vi "Autonics_Hall_GMR_Vector.vi"() -> ()   [LabVIEW 2018]
uses:
  <vilib>/Platform/NI_3dgraph.lvlib
  <vilib>/Utility/file.llb/Write To Spreadsheet File (DBL).vi
  <vilib>/DAQmx/create/channels.llb/DAQmx Create Channel (DO-Digital Output).vi
  <vilib>/DAQmx/write.llb/DAQmx Write (Digital 1D Bool 1Chan 1Samp).vi
  <vilib>/DAQmx/read.llb/DAQmx Read (Analog 2D DBL NChan NSamp).vi
  <vilib>/DAQmx/configure/timing.llb/DAQmx Timing (Sample Clock).vi
  <vilib>/DAQmx/create/channels.llb/DAQmx Create Channel (AI-Voltage-Basic).vi
  <resource>/objmgr/daqmx.rc
  <vilib>/Math Plots/3D Math Plots/3D Quiver/3D Quiver Datatype/3D Quiver Datatype.lvclass
  <vilib>/Math Plots/3D Math Plots/3D Quiver/3D Quiver Datatype/Public/Plot Helper (Vector).vi
  <vilib>/Analysis/Matrix/NI_Matrix.lvlib
  <vilib>/Utility/file.llb/Read From Spreadsheet File (DBL).vi
  <vilib>/Analysis/Matrix/Numeric/Multiply/Multiply - R,RM.vi
  <vilib>/Analysis/Matrix/Numeric/Multiply/Multiply - RM,R.vi
  <vilib>/Math Plots/2D Math Plots/2D Feather/2D Feather Datatype/2D Feather Datatype.lvclass
  <vilib>/Math Plots/2D Math Plots/2D Feather/2D Feather Datatype/Public/Plot Helper (Vector).vi
  <vilib>/Instr/_visa.llb/VISA Configure Serial Port (Instr).vi
  <vilib>/Math Plots/3D Math Plots/3D Quiver/3D Quiver XCtrl/3D Quiver.xctl
  <vilib>/Math Plots/2D Math Plots/2D Feather/2D Feather XCtrl/2D Feather.xctl
panel:
  out "2D Feather":refnum<class "2D Plot Datatype.lvclass">[](xcontrol)
  in  "GMR":refnum<k7>(container)
  in  "Z Length":dbl=2.0
  out "X Length":dbl=50.0
  out "X_Z_Scale":sgl=111.11112
  in  "Invert ?":bool
  out "Time Step":u32
  in  "Open":bool
  out "3D Vector":refnum<class "3D Plot Datatype.lvclass">[](xcontrol)
  in  "Scan Distance":dbl=50.0
  in  "Multiplier":dbl=10.0
  in  "Save Button":bool
  in  "No Save":bool
  in  "Save/Open Link":path
  in  "ViewMode":i32(ring) items=["cwViewXYPlane", "cwViewXZPlane", "cwViewYZPlane", "cwViewUserDefined"]
  in  "Back data":bool
  in  "Data Type":u16(ring) items=["Normal", "dX", "dY"]
  in  "Scan Channel":fxp<+,8,8>
  in  "Scan Channel Control":tag="Dev3/port0/line0:7"
  in  "Sampling Rate(Hz)":dbl=15000.0
  in  "Samples per Channels":i32=1000
  in  "Min Volts":dbl=-10.0 format="%0.2f"
  in  "Max Volts":dbl=10.0 format="%0.2f"
  in  "Channels":tag="Dev3/ai0:63"
  in  "Scan Step (mm)":dbl=1.0
  in  "Scan":bool
  in  "Plot style":i32(ring)=5 items=["cwLine"=1, "cwPoint"=2, "cwLinePoint"=3, "cwHiddenLine"=4, "cwSurface"=5, "cwSurfaceLine"=6, "cwSurfaceNormal"=7, "cwContourLine"=8, "cwSurfaceContour"=9]
  in  "Hall":refnum<k7>(container)
  in  "Flow control":u16(ring) items=["None", "XON/XOFF", "RTS/CTS", "XON/XOFF & RTS/CTS", "DTR/DSR", "XON/XOFF & DTR/DSR"]
  in  "Stop bits":u16(ring)=10 items=["1.0"=10, "1.5"=15, "2.0"=20]
  in  "Parity":dbl
  in  "Data bits":u16=8 min=5 max=8 step=1
  in  "Baud Rate":u32=57600
  in  "COM Port":refnum<visa-resource-name>="COM3"
  in  "Travel per Pulse (mm)":dbl=0.002
  in  "Speed (mm/s)":dbl=5.0
  out "Current  Position (mm)":dbl format="%#_4g"
  in  "Move Distance (mm)":dbl=1.0
  in  "Stop Scan":bool
  in  "Stop":bool
  in  "Home":bool
  in  "Right":bool
  in  "Left":bool
  # "SCANER CONTROL"
  # "CRACKS INSPECTION"
  # "COM Setting"
  # "CHANNELS"
  # "TIMING"
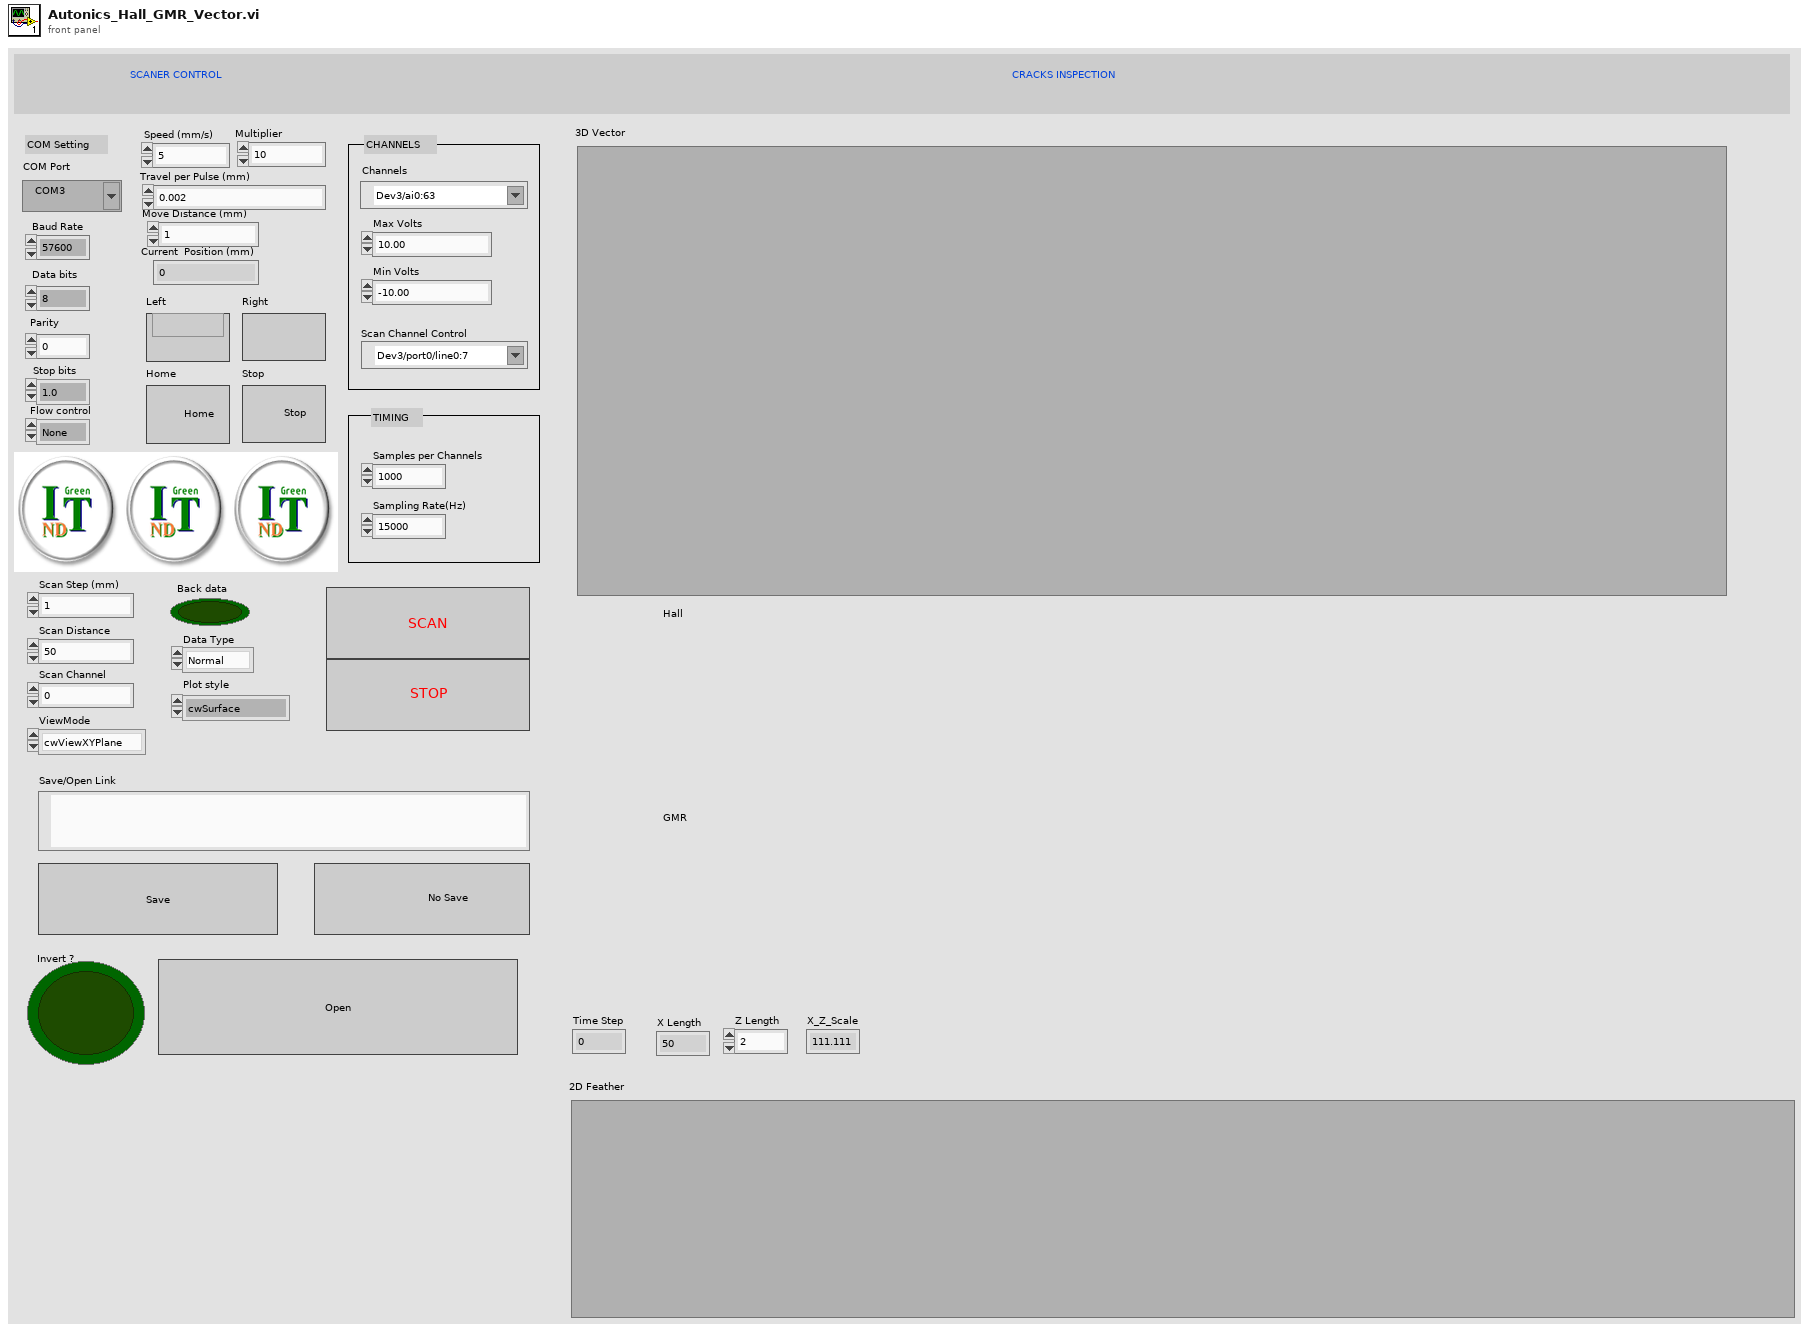
[diagram p1: front panel]
types:
  T1 = typedef "NI_Matrix.lvlib/RealMatrix.ctl" = dbl[][]
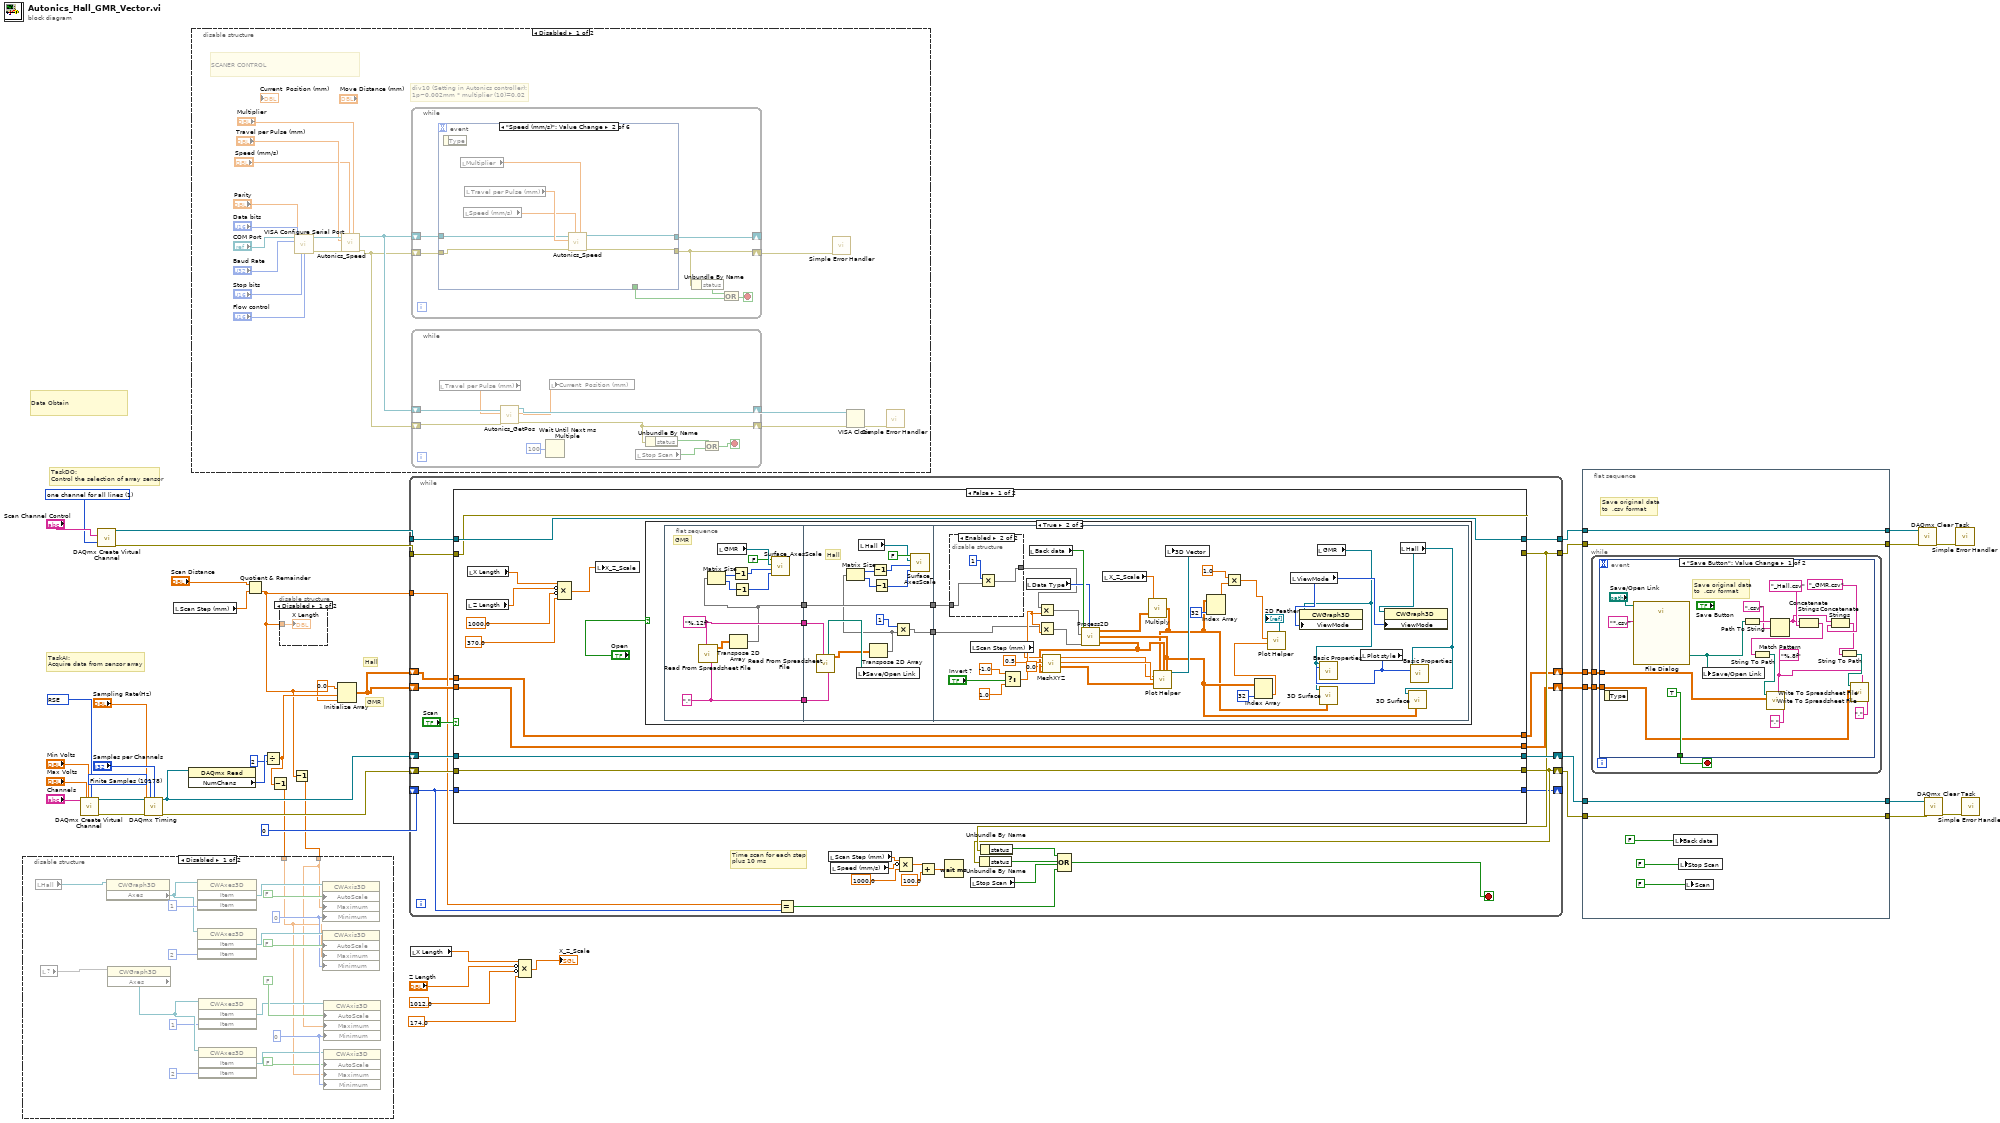
[diagram p0: block diagram]
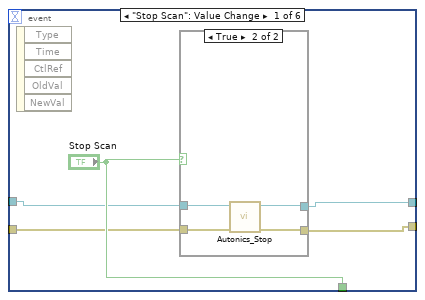
[diagram p4: hidden frame]
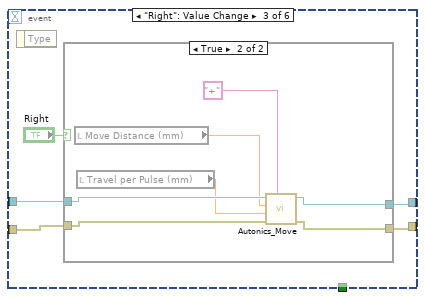
[diagram p6: hidden frame]
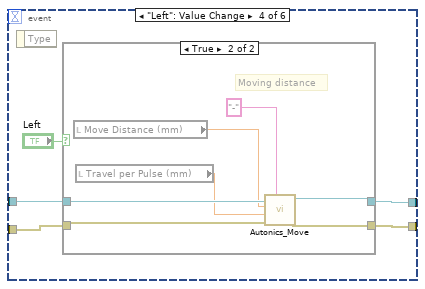
[diagram p8: hidden frame]
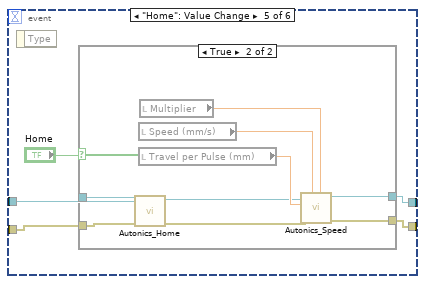
[diagram p10: hidden frame]
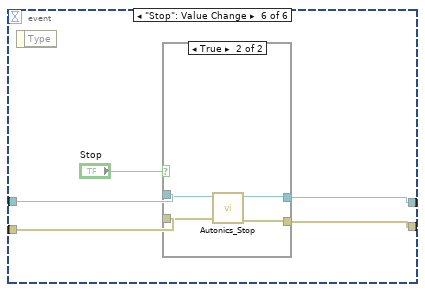
[diagram p12: hidden frame]
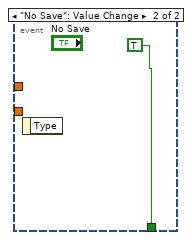
[diagram p15: hidden frame]
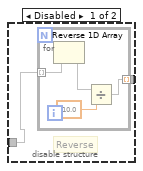
[diagram p17: hidden frame]
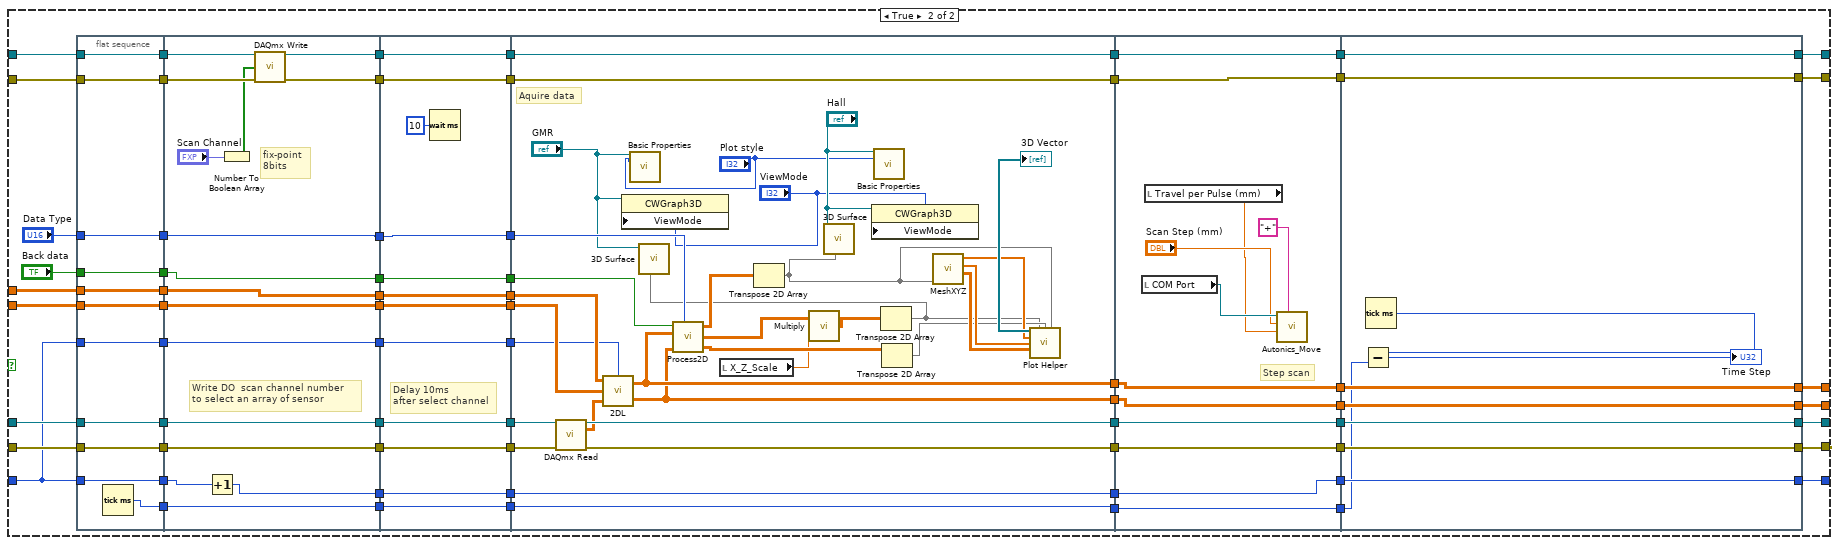
[diagram p18: hidden frame]
diagram:
  w20 = 10083 items=["default"=-1, "RSE"=10083, "NRSE"=10078, "Differential"=10106, "Pseudodifferential"=12529] ("input terminal configuration")
  w28 = 1 items=["one channel for each line", "one channel for all lines"] ("line grouping")
  w34 = 10178 items=["Finite Samples"=10178, "Continuous Samples"=10123, "Hardware Timed Single Point"=12522] ("sample mode")
  # "GMR"
  # "Hall"
  # "TaskAI:\nAcquire data from sensor array"
  # "TaskDO: \nControl the selection of array sensor"
  # "Data Obtain"
  n1 = call-poly <vilib>:"DAQmx Create Virtual Channel.vi"("maximum value"="Max Volts", "minimum value"="Min Volts", "input terminal configuration"=w20, "physical channels"="Channels") -> ("task out"=w43:refnum<k21>, "error out"=w42:errorcluster)  [unwired: 10 in]
  n2 = call-poly <vilib>:"DAQmx Create Virtual Channel.vi"("lines"="Scan Channel Control", "line grouping"=w28) -> ("task out"=w27:refnum<k21>, "error out"=w26:errorcluster)  [unwired: 12 in]
  n3 = call-poly <vilib>:"DAQmx Timing.vi"("task/channels in"=w43, "sample mode"=w34, "samples per channel"="Samples per Channels", "rate"="Sampling Rate(Hz)", "error in"=w42) -> ("task out"=w18:refnum<k21>, "error out"=w36:errorcluster)  [unwired: 9 in]
  n4 = local read "Scan Step (mm)"() -> (w17:dbl)
  n5 = property class="DAQmx Read"(reference=w18) -> ("NumChans"=w13:u32)  [unwired: 1 in, 2 out]
  n6 = disable-structure shown="Disabled" {
    frame Disabled {
      # "div10 (Setting in Autonics controller):\n1p~0.002mm * multiplier (10)=0.02"
      # "SCANER CONTROL"
      n7 = call-poly "VISA Configure Serial Port"("VISA resource name"="COM Port", "baud rate (9600)"="Baud Rate", "data bits (8)"="Data bits", "parity (0:none)"="Parity", "stop bits (10: 1 bit)"="Stop bits", "flow control (0:none)"="Flow control") -> ("VISA resource name out"=w48:refnum<visa-resource-name>, "error out"=w47:errorcluster)  [unwired: 8 in]
      n8 = call "Autonics_Speed.vi"("Multiplier"="Multiplier", "Speed (mm/s)"="Speed (mm/s)", "error in (no error)"=w47, "Travel per  Pulse"="Travel per Pulse (mm)", "VISA resource name"=w48) -> ("error out"=w49:errorcluster, "VISA resource name out"=w50:refnum<visa-resource-name>)  [unwired: 5 in]
      n9 = while {
        shift-right: [w77] -> _
        shift-left: w50 -> [w76]
        shift-right: [w73] -> w53
        shift-left: w49 -> [w75]
        stop <- w72 stop-if-true
        n10 = event shown="[1] \"Speed (mm/s)\": Value Change" {
          selector: _ -> [_ _ _ _ _ _]
          dyn-events: _ -> [_ _ _ _ _ _]
          timeout: _ -> [_ _ _ _ _ _]
          tunnel: w76 -> [w81 w94 w98 w112 w128 w142]
          tunnel: w75 -> [w80 w93 w97 w111 w127 w141]
          tunnel: [w79 w92 w100 w114 w125 w144] -> w77
          tunnel: [w78 w91 w99 w113 w124 w143] -> w73
          tunnel: ["Stop Scan" _ _ _ _ _] -> w71
          event "Stop Scan": Value Change {
            n11 = event-data() -> ()  [unwired: 1 in, 5 out]
            n12 = case shown="True" "Stop Scan" {
              tunnel: [w84 w87] -> w79
              tunnel: [w83 w88] -> w78
              tunnel: w81 -> [w84 w86]
              tunnel: w80 -> [w83 w85]
              frame False {
              }
              frame True {
                n13 = call "Autonics_Stop.vi"("error in (no error)"=w85, "VISA resource name"=w86) -> ("error out"=w88:errorcluster, "VISA resource name out"=w87:refnum<visa-resource-name>)  [unwired: 8 in]
              }
            }
          }
          event "Speed (mm/s)": Value Change {
            n14 = event-data() -> ()  [unwired: 1 in, 1 out]
            n15 = local read "Multiplier"() -> (w89:dbl)
            n16 = local read "Speed (mm/s)"() -> (w90:dbl)
            n17 = local read "Travel per Pulse (mm)"() -> (w95:dbl)
            n18 = call "Autonics_Speed.vi"("Multiplier"=w89, "Speed (mm/s)"=w90, "error in (no error)"=w93, "Travel per  Pulse"=w95, "VISA resource name"=w94) -> ("error out"=w91:errorcluster, "VISA resource name out"=w92:refnum<visa-resource-name>)  [unwired: 5 in]
          }
          event "Right": Value Change {
            n19 = event-data() -> ()  [unwired: 1 in, 1 out]
            n20 = case shown="True" "Right" {
              tunnel: [w101 w107] -> w100
              tunnel: [w102 w106] -> w99
              tunnel: w98 -> [w101 w109]
              tunnel: w97 -> [w102 w108]
              frame False {
              }
              frame True {
                n21 = local read "Move Distance (mm)"() -> (w105:dbl)
                n22 = local read "Travel per Pulse (mm)"() -> (w104:dbl)
                n23 = call "Autonics_Move.vi"("Direction (+)"="+", "error in (no error)"=w108, "Travel per Pulse (mm)"=w104, "Move Distance (mm)"=w105, "VISA resource name"=w109) -> ("error out"=w106:errorcluster, "VISA resource name out"=w107:refnum<visa-resource-name>)  [unwired: 5 in]
              }
            }
          }
          event "Left": Value Change {
            n24 = event-data() -> ()  [unwired: 1 in, 1 out]
            n25 = case shown="True" "Left" {
              tunnel: [w116 w121] -> w114
              tunnel: [w115 w120] -> w113
              tunnel: w112 -> [w116 w123]
              tunnel: w111 -> [w115 w122]
              frame False {
              }
              frame True {
                # "Moving distance"
                n26 = local read "Move Distance (mm)"() -> (w118:dbl)
                n27 = local read "Travel per Pulse (mm)"() -> (w117:dbl)
                n28 = call "Autonics_Move.vi"("Direction (+)"="-", "error in (no error)"=w122, "Travel per Pulse (mm)"=w117, "Move Distance (mm)"=w118, "VISA resource name"=w123) -> ("error out"=w120:errorcluster, "VISA resource name out"=w121:refnum<visa-resource-name>)  [unwired: 5 in]
              }
            }
          }
          event "Home": Value Change {
            n29 = event-data() -> ()  [unwired: 1 in, 1 out]
            n30 = case shown="True" "Home" {
              tunnel: [w130 w132] -> w125
              tunnel: [w129 w131] -> w124
              tunnel: w128 -> [w130 w139]
              tunnel: w127 -> [w129 w138]
              frame False {
              }
              frame True {
                n31 = call "Autonics_Home.vi"("error in (no error)"=w138, "VISA resource name"=w139) -> ("error out"=w133:errorcluster, "VISA resource name out"=w134:refnum<visa-resource-name>)  [unwired: 8 in]
                n32 = local read "Speed (mm/s)"() -> (w136:dbl)
                n33 = local read "Travel per Pulse (mm)"() -> (w137:dbl)
                n34 = local read "Multiplier"() -> (w135:dbl)
                n35 = call "Autonics_Speed.vi"("Multiplier"=w135, "Speed (mm/s)"=w136, "error in (no error)"=w133, "Travel per  Pulse"=w137, "VISA resource name"=w134) -> ("error out"=w131:errorcluster, "VISA resource name out"=w132:refnum<visa-resource-name>)  [unwired: 5 in]
              }
            }
          }
          event "Stop": Value Change {
            n36 = event-data() -> ()  [unwired: 1 in, 1 out]
            n37 = case shown="True" "Stop" {
              tunnel: [w146 w147] -> w144
              tunnel: [w145 w150] -> w143
              tunnel: w142 -> [w146 w149]
              tunnel: w141 -> [w145 w148]
              frame False {
              }
              frame True {
                n38 = call "Autonics_Stop.vi"("error in (no error)"=w148, "VISA resource name"=w149) -> ("error out"=w150:errorcluster, "VISA resource name out"=w147:refnum<visa-resource-name>)  [unwired: 8 in]
              }
            }
          }
        }
        n39 = Unbundle By Name(w73) -> ("status"=w74:bool)
        n40 = Compound Arithmetic op=OR(w74, w71) -> (w72:bool)
      }
      n41 = while {
        shift-right: [w64] -> w52
        shift-left: w50 -> [w66]
        shift-right: [w63] -> w51
        shift-left: w49 -> [w65]
        stop <- w67 stop-if-true
        n42 = local read "Travel per Pulse (mm)"() -> (w62:dbl)
        n43 = call "Autonics_GetPos.vi"("error in (no error)"=w65, "Travel per Pulse (mm)"=w62, "VISA resource name"=w66) -> ("error out"=w63:errorcluster, "Current  Position (mm)"=w61:dbl, "VISA resource name out"=w64:refnum<visa-resource-name>)  [unwired: 6 in]
        n44 = Wait Until Next ms Multiple(millisecond multiple=u32 100) -> ()  [unwired: 1 out]
        n45 = local write "Current  Position (mm)"(w61) -> ()
        n46 = local read "Stop Scan"() -> (w68:bool)
        n47 = Unbundle By Name(w63) -> ("status"=w69:bool)
        n48 = Compound Arithmetic op=OR(w69, w68) -> (w67:bool)
      }
      n49 = call <vilib>:"Simple Error Handler.vi"("error in (no error)"=w53) -> ()  [unwired: 4 in, 5 out]
      n50 = VISA Close(VISA resource name=w52, error in (no error)=w51) -> (error out=w56:errorcluster)
      n51 = call <vilib>:"Simple Error Handler.vi"("error in (no error)"=w56) -> ()  [unwired: 4 in, 5 out]
    }
    frame Enabled {
    }
  }
  n52 = Quotient & Remainder(x="Scan Distance", y=w17) -> (floor(x/y)=w7:dbl)  [unwired: 1 out]
  n53 = Divide(x=w13, y=u32 2) -> (x/y=w9:dbl)
  n54 = Decrement(x=w9) -> (x-1=w10:dbl)
  n55 = disable-structure shown="Disabled" {
    disable-tunnel: w7 -> [w151 _]
    frame Disabled {
      "X Length" <- w151
    }
    frame Enabled {
    }
  }
  n56 = Decrement(x=w7) -> (x-1=w8:dbl)
  n57 = disable-structure shown="Disabled" {
    disable-tunnel: w10 -> [w153 _]
    disable-tunnel: w8 -> [w152 _]
    frame Disabled {
      w162 = 0
      w163 = 0
      n58 = local read "Hall"() -> (w171:refnum<k7>)
      n59 = local read item#-1() -> (w154)
      n60 = property class="CWGraph3D"(reference=w171) -> ("Axes"=w164:refnum<k7>)  [unwired: 1 in, 2 out]
      n61 = property class="CWGraph3D"(reference=w154) -> ("Axes"=w161:refnum<k7>)  [unwired: 1 in, 2 out]
      n62 = invoke class="CWAxes3D" method="Item"(reference=w164, "Item"=1) -> ("Item"=w170:refnum<k7>)  [unwired: 2 in, 3 out]
      n63 = invoke class="CWAxes3D" method="Item"(reference=w164, "Item"=2) -> ("Item"=w165:refnum<k7>)  [unwired: 2 in, 3 out]
      n64 = invoke class="CWAxes3D" method="Item"(reference=w161, "Item"=1) -> ("Item"=w155:refnum<k7>)  [unwired: 2 in, 3 out]
      n65 = invoke class="CWAxes3D" method="Item"(reference=w161, "Item"=2) -> ("Item"=w160:refnum<k7>)  [unwired: 2 in, 3 out]
      n66 = property class="CWAxis3D"(reference=w170, "AutoScale"=FALSE, "Maximum"=w152, "Minimum"=w163) -> ()  [unwired: 1 in, 2 out]
      n67 = property class="CWAxis3D"(reference=w165, "AutoScale"=FALSE, "Maximum"=w153, "Minimum"=w163) -> ()  [unwired: 1 in, 2 out]
      n68 = property class="CWAxis3D"(reference=w155, "AutoScale"=FALSE, "Maximum"=w152, "Minimum"=w162) -> ()  [unwired: 1 in, 2 out]
      n69 = property class="CWAxis3D"(reference=w160, "AutoScale"=FALSE, "Maximum"=w153, "Minimum"=w162) -> ()  [unwired: 1 in, 2 out]
    }
    frame Enabled {
    }
  }
  n70 = Initialize Array(0.0 ("element"), w9, w7) -> (w14:dbl[][])
  n71 = while {
    shift-right: [w172] -> w1
    shift-left: w14 -> [w197]
    shift-right: [w195] -> w33
    shift-left: w18 -> [w196]
    shift-right: [w187] -> w31
    shift-left: w36 -> [w198]
    tunnel: w27 -> [w191]
    tunnel: w26 -> [w190]
    tunnel: [w189] -> w24
    tunnel: [w188] -> w23
    shift-right: [w178] -> _
    shift-left: 0 -> [w176]
    tunnel: w7 -> [w177]
    shift-right: [w173] -> w11
    shift-left: w14 -> [w174]
    stop <- w194 stop-if-true
    # "Time scan for each step\nplus 10 ms"
    n72 = case shown="False" "Scan" {
      tunnel: w196 -> [w211 w348]
      tunnel: w198 -> [w210 w347]
      tunnel: w197 -> [w206 w346]
      tunnel: [w211 w343] -> w195
      tunnel: [w210 w342] -> w187
      tunnel: [w205 w309] -> w173
      tunnel: w191 -> [w209 w341]
      tunnel: w190 -> [w208 w340]
      tunnel: [w209 w337] -> w189
      tunnel: [w208 w336] -> w188
      tunnel: [w207 w319] -> w178
      tunnel: w176 -> [w207 w312]
      tunnel: w174 -> [w205 w313]
      tunnel: [w206 w307] -> w172
      frame False {
        n73 = local read "Z Length"() -> (w203:dbl)
        n74 = local read "X Length"() -> (w202:dbl)
        n75 = Compound Arithmetic op=MULTIPLY(w202, invert w203, invert 1000.0 ("value"), 370.0 ("value")) -> (w199:dbl)
        n76 = local write "X_Z_Scale"(w199) -> ()
        n77 = case shown="True" "Open" {
          frame False {
          }
          frame True {
            n78 = flat-sequence {
              tunnel: [w218] -> w215
              tunnel: [w226] -> w213
              tunnel: [w225] -> w212
              tunnel: [w240] -> w216
              tunnel: w215 -> [w240]
              tunnel: [w230] -> w214
              tunnel: w213 -> [w239]
              tunnel: w212 -> [w238]
              tunnel: w216 -> [w257]
              tunnel: w214 -> [w246]
              frame #0 {
                w226 = "," ("delimiter (\\t)")
                w225 = "%.12f" ("format (%.3f)")
                # "GMR"
                n79 = call-poly <vilib>:"Read From Spreadsheet File.vi"("delimiter (\\t)"=w226, "format (%.3f)"=w225) -> ("all rows"=w217:dbl[][])  [unwired: 5 in, 4 out]
                n80 = local read "GMR"() -> (w221:refnum<k7>)
                n81 = Transpose 2D Array(2D array=w217) -> (transposed array=w218:dbl[][])
                n82 = Matrix Size(0:w218) -> (1:w219:i32, 2:w223:i32)
                n83 = Decrement(x=w219) -> (x-1=w222:i32)
                n84 = Decrement(x=w223) -> (x-1=w224:i32)
                n85 = call "Surface_AxesScale.vi"("Y-axis Max"=w224, "X-axis max"=w222, "3D Surface"=w221, "Auto Scale"=FALSE) -> ()  [unwired: 8 in]
              }
              frame #1 {
                # "Hall"
                n86 = call-poly <vilib>:"Read From Spreadsheet File.vi"("delimiter (\\t)"=w239, "format (%.3f)"=w238) -> ("all rows"=w228:dbl[][], "new file path (Not A Path if cancelled)"=w237:path)  [unwired: 5 in, 3 out]
                n87 = local write "Save/Open Link"(w237) -> ()
                n88 = local read "Hall"() -> (w234:refnum<k7>)
                n89 = Transpose 2D Array(2D array=w228) -> (transposed array=w227:dbl[][])
                n90 = Matrix Size(0:w227) -> (1:w236:i32, 2:w232:i32)
                n91 = Decrement(x=w236) -> (x-1=w233:i32)
                n92 = Decrement(x=w232) -> (x-1=w231:i32)
                n93 = Multiply(x=1, y=w227) -> (x*y=w230:dbl[][])
                n94 = call "Surface_AxesScale.vi"("Y-axis Max"=w231, "X-axis max"=w233, "3D Surface"=w234, "Auto Scale"=FALSE) -> ()  [unwired: 8 in]
              }
              frame #2 {
                n95 = disable-structure shown="Enabled" {
                  disable-tunnel: w257 -> [w276 w283]
                  disable-tunnel: [w275 w282] -> w247
                  frame Disabled {
                    # "Reverse"
                    n96 = for {
                      tunnel: w276 -> [w280] mode=indexing
                      tunnel: [w277] -> w275 mode=indexing
                      n97 = Reverse 1D Array(array=w280) -> (reversed array=w278:dbl[])
                      n98 = Divide(x=w278, y=-10.0 ("t")) -> (x/y=w277:dbl[])
                    }
                  }
                  frame Enabled {
                    n99 = Multiply(x=1, y=w283) -> (x*y=w282:dbl[][])
                  }
                }
                n100 = local read "Scan Step (mm)"() -> (w260:dbl)
                n101 = Select(t=-1.0, s="Invert ?", f=1.0) -> (s? t:f=w268:dbl)
                n102 = local read "Data Type"() -> (w261:u16)
                n103 = local read "Back data"() -> (w262:bool)
                n104 = Multiply(x=w247, y=w268) -> (x*y=w255:dbl[][])
                n105 = Multiply(x=w246, y=w268) -> (x*y=w267:dbl[][])
                n106 = call "Process2D.vi"("Back Data"=w262, "Matrix X"=w255, "Matrix Y"=w267, "Data Type"=w261) -> ("Out Matrix X"=w244:T1, "Out Matrix Y"=w245:T1, "Out Matrix Z (zeros)"=w256:T1)  [unwired: 1 in]
                n107 = call "MeshXYZ.vi"("Input Matrix)"=w256, "Z- Lift-off"=0.0, "del Y"=0.5, "del X"=w260) -> ("Mesh Z (Matrix)"=w243:dbl[][], "Mesh Y (Array)"=w274:dbl[], "Mesh X (Array)"=w273:dbl[])  [unwired: 5 in]
                n108 = local read "X_Z_Scale"() -> (w258:sgl)
                n109 = call-poly <vilib>:"Multiply.vi"("Real Matrix A"=w244, "Real Scalar c"=w258) -> ("c * A"=w242:T1)
                n110 = call-poly <vilib>:"Plot Helper.vi"("Nx matrix"=w242, "Ny matrix"=w256, "Nz matrix"=w245, "x vector"=w273, "y vector"=w274, "z matrix"=w243) -> ("3D Plot lvclass Array out"=w272:refnum<class "3D Plot Datatype.lvclass">[])  [unwired: 3 in, 6 out]
                n111 = local write "3D Vector"(w272) -> ()
                n112 = Index Array(array=w242, index (col)=32 ("disabled index (col)")) -> (element=w249:dbl[])  [unwired: 1 in]
                n113 = Multiply(x=1.0, y=w249) -> (x*y=w248:dbl[])
                n114 = Index Array(array=w245, index (col)=32 ("disabled index (col)")) -> (element=w251:dbl[])  [unwired: 1 in]
                n115 = call-poly <vilib>:"Plot Helper.vi"("y vector"=w251, "x vector"=w248) -> ("2D Plot Class Obj Array out"=→"2D Feather":refnum<class "2D Plot Datatype.lvclass">[])  [unwired: 2 in, 7 out]
                n116 = local read "ViewMode"() -> (w265:i32)
                n117 = local read "GMR"() -> (w263:refnum<k7>)
                n118 = property class="CWGraph3D"(reference=w263, "ViewMode"=w265) -> ()  [unwired: 1 in, 2 out]
                n119 = call <vilib>:"3D Surface.vi"("z matrix"=w242, "3D graph"=w263) -> ()  [unwired: 8 in, 2 out]
                n120 = local read "Plot style"() -> (w266:i32)
                n121 = call <vilib>:"Basic Properties.vi"("3D graph"=w263, "plot style"=w266) -> ()  [unwired: 12 in, 2 out]
                n122 = local read "Hall"() -> (w264:refnum<k7>)
                n123 = property class="CWGraph3D"(reference=w264, "ViewMode"=w265) -> ()  [unwired: 1 in, 2 out]
                n124 = call <vilib>:"3D Surface.vi"("z matrix"=w245, "3D graph"=w264) -> ()  [unwired: 8 in, 2 out]
                n125 = call <vilib>:"Basic Properties.vi"("3D graph"=w264, "plot style"=w266) -> ()  [unwired: 12 in, 2 out]
              }
            }
          }
        }
      }
      frame True {
        n126 = flat-sequence {
          tunnel: w312 -> [w350]
          tunnel: w313 -> [w351]
          tunnel: w312 -> [w352]
          tunnel: "Data Type" -> [w353]
          tunnel: "Back data" -> [w354]
          tunnel: w340 -> [w355]
          tunnel: w341 -> [w356]
          tunnel: w346 -> [w357]
          tunnel: w347 -> [w358]
          tunnel: w348 -> [w359]
          tunnel: [w359] -> w305
          tunnel: [w358] -> w304
          tunnel: [w357] -> w303
          tunnel: [w356] -> w302
          tunnel: [w355] -> w301
          tunnel: [w354] -> w300
          tunnel: [w353] -> w299
          tunnel: [w352] -> w298
          tunnel: [w351] -> w297
          tunnel: [w350] -> w296
          tunnel: [w349] -> w292
          tunnel: [w375] -> w335
          tunnel: [w374] -> w333
          tunnel: [w373] -> w331
          tunnel: [w370] -> w329
          tunnel: [w369] -> w327
          tunnel: [w366] -> w323
          tunnel: [w365] -> w322
          tunnel: [w363] -> w316
          tunnel: [w362] -> w314
          tunnel: [w361] -> w311
          tunnel: w305 -> [w375]
          tunnel: w304 -> [w374]
          tunnel: w303 -> [w373]
          tunnel: w302 -> [w372]
          tunnel: w301 -> [w371]
          tunnel: w300 -> [w366]
          tunnel: w299 -> [w365]
          tunnel: w298 -> [w364]
          tunnel: w297 -> [w362]
          tunnel: w296 -> [w361]
          tunnel: [w360] -> w293
          tunnel: w292 -> [w360]
          tunnel: w335 -> [w387]
          tunnel: [w387] -> w334
          tunnel: w333 -> [w386]
          tunnel: [w386] -> w332
          tunnel: w331 -> [w385]
          tunnel: [w385] -> w330
          tunnel: w329 -> [w384]
          tunnel: [w384] -> w328
          tunnel: w327 -> [w383]
          tunnel: [w383] -> w326
          tunnel: [w381] -> w324
          tunnel: w323 -> [w381]
          tunnel: w322 -> [w380]
          tunnel: [w380] -> w320
          tunnel: [w379] -> w317
          tunnel: w316 -> [w379]
          tunnel: [w378] -> w315
          tunnel: w314 -> [w378]
          tunnel: w311 -> [w377]
          tunnel: [w377] -> w310
          tunnel: [w376] -> w294
          tunnel: w293 -> [w376]
          tunnel: [w417] -> w345
          tunnel: [w416] -> w344
          tunnel: w334 -> [w419]
          tunnel: w332 -> [w418]
          tunnel: w330 -> [w409]
          tunnel: [w415] -> w339
          tunnel: w328 -> [w415]
          tunnel: [w414] -> w338
          tunnel: w326 -> [w414]
          tunnel: w324 -> [w402]
          tunnel: w320 -> [w401]
          tunnel: [w412] -> w318
          tunnel: w317 -> [w412]
          tunnel: w315 -> [w410]
          tunnel: w310 -> [w408]
          tunnel: [w407] -> w308
          tunnel: [w406] -> w306
          tunnel: [w395] -> w295
          tunnel: w294 -> [w395]
          tunnel: w345 -> [w431]
          tunnel: w344 -> [w430]
          tunnel: w339 -> [w429]
          tunnel: w338 -> [w428]
          tunnel: w318 -> [w427]
          tunnel: w308 -> [w426]
          tunnel: w306 -> [w425]
          tunnel: w295 -> [w424]
          tunnel: [w431] -> w291
          tunnel: [w430] -> w290
          tunnel: [w429] -> w289
          tunnel: [w428] -> w288
          tunnel: [w427] -> w287
          tunnel: [w426] -> w286
          tunnel: [w425] -> w285
          tunnel: [w424] -> w284
          tunnel: [w435] -> w307
          tunnel: [w436] -> w309
          tunnel: [w437] -> w319
          tunnel: [w438] -> w336
          tunnel: [w439] -> w337
          tunnel: [w440] -> w342
          tunnel: [w441] -> w343
          tunnel: w291 -> [w441]
          tunnel: w290 -> [w440]
          tunnel: w289 -> [w439]
          tunnel: w288 -> [w438]
          tunnel: w287 -> [w437]
          tunnel: w286 -> [w436]
          tunnel: w285 -> [w435]
          tunnel: w284 -> [w433]
          frame #0 {
            n127 = Tick Count (ms)() -> (millisecond timer value=w349:u32)
          }
          frame #1 {
            # "fix-point\n8bits"
            # "Write DO  scan channel number\nto select an array of sensor"
            n128 = Increment(x=w364) -> (x+1=w363:i32)
            n129 = Number To Boolean Array(number="Scan Channel") -> (Boolean array=w367:bool[])
            n130 = call-poly <vilib>:"DAQmx Write.vi"("task/channels in"=w372, "data"=w367, "error in"=w371) -> ("task out"=w370:refnum<k21>, "error out"=w369:errorcluster)  [unwired: 10 in, 1 out]
          }
          frame #2 {
            # "Delay 10ms\nafter select channel"
            n131 = Wait (ms)(milliseconds to wait=u32 10) -> ()  [unwired: 1 out]
          }
          frame #3 {
            # "Aquire data"
            n132 = call-poly <vilib>:"DAQmx Read.vi"("task/channels in"=w419, "error in"=w418) -> ("task out"=w417:refnum<k21>, "data"=w411:dbl[][], "error out"=w416:errorcluster)  [unwired: 11 in]
            n133 = call "2DL.vi"("Insert Colum"=w408, "Input Matrix"=w411, "Input Array Y"=w409, "Input Array X"=w410) -> ("Out Array Y"=w406:dbl[][], "Out Array X"=w407:dbl[][])
            n134 = property class="CWGraph3D"(reference="GMR", "ViewMode"="ViewMode") -> ()  [unwired: 1 in, 2 out]
            n135 = call <vilib>:"Basic Properties.vi"("3D graph"="GMR", "plot style"="Plot style") -> ()  [unwired: 12 in, 2 out]
            n136 = call "Process2D.vi"("Back Data"=w402, "Matrix X"=w407, "Matrix Y"=w406, "Data Type"=w401) -> ("Out Matrix X"=w403:T1, "Out Matrix Y"=w391:T1, "Out Matrix Z (zeros)"=w405:T1)  [unwired: 1 in]
            n137 = local read "X_Z_Scale"() -> (w390:sgl)
            n138 = Transpose 2D Array(2D array=w403) -> (transposed array=w394:T1)
            n139 = call-poly <vilib>:"Multiply.vi"("Real Scalar c"=w390, "Real Matrix A"=w391) -> ("A * c"=w389:T1)
            n140 = call <vilib>:"3D Surface.vi"("z matrix"=w394, "3D graph"="Hall") -> ()  [unwired: 8 in, 2 out]
            n141 = property class="CWGraph3D"(reference="Hall", "ViewMode"="ViewMode") -> ()  [unwired: 1 in, 2 out]
            n142 = call <vilib>:"Basic Properties.vi"("3D graph"="Hall", "plot style"="Plot style") -> ()  [unwired: 12 in, 2 out]
            n143 = Transpose 2D Array(2D array=w389) -> (transposed array=w392:T1)
            n144 = call <vilib>:"3D Surface.vi"("z matrix"=w392, "3D graph"="GMR") -> ()  [unwired: 8 in, 2 out]
            n145 = Transpose 2D Array(2D array=w405) -> (transposed array=w393:T1)
            n146 = call "MeshXYZ.vi"("Input Matrix)"=w394) -> ("Mesh Z (Matrix)"=w400:dbl[][], "Mesh Y (Array)"=w399:dbl[], "Mesh X (Array)"=w398:dbl[])  [unwired: 8 in]
            n147 = call-poly <vilib>:"Plot Helper.vi"("Nx matrix"=w392, "Ny matrix"=w393, "Nz matrix"=w394, "x vector"=w398, "y vector"=w399, "z matrix"=w400) -> ("3D Plot lvclass Array out"=→"3D Vector":refnum<class "3D Plot Datatype.lvclass">[])  [unwired: 3 in, 6 out]
          }
          frame #4 {
            # "Step scan"
            n148 = local read "COM Port"() -> (w423:refnum<visa-resource-name>)
            n149 = local read "Travel per Pulse (mm)"() -> (w421:dbl)
            n150 = call "Autonics_Move.vi"("Direction (+)"="+", "Travel per Pulse (mm)"=w421, "Move Distance (mm)"="Scan Step (mm)", "VISA resource name"=w423) -> ()  [unwired: 6 in, 2 out]
          }
          frame #5 {
            n151 = Tick Count (ms)() -> (millisecond timer value=w434:u32)
            n152 = Subtract(x=w434, y=w433) -> (x-y=→"Time Step":u32)
          }
        }
      }
    }
    n153 = Equal?(x=w177, y=w176) -> (x = y?=w175:bool)
    n154 = local read "Scan Step (mm)"() -> (w184:dbl)
    n155 = local read "Speed (mm/s)"() -> (w183:dbl)
    n156 = Compound Arithmetic op=MULTIPLY(w184, invert w183, 1000.0 ("value")) -> (w181:dbl)
    n157 = Add(x=w181, y=100.0) -> (x+y=w179:dbl)
    n158 = Wait (ms)(milliseconds to wait=w179) -> ()  [unwired: 1 out]
    n159 = local read "Stop Scan"() -> (w192:bool)
    n160 = Unbundle By Name(w187) -> ("status"=w185:bool)
    n161 = Unbundle By Name(w188) -> ("status"=w186:bool)
    n162 = Compound Arithmetic op=OR(w186, w185, w192, w175) -> (w194:bool)
  }
  n163 = local read "X Length"() -> (w6:dbl)
  n164 = Compound Arithmetic op=MULTIPLY(w6, invert "Z Length", invert 1012.0 ("value"), 174.0 ("value")) -> (→"X_Z_Scale":dbl)
  n165 = flat-sequence {
    tunnel: w33 -> [w450]
    tunnel: [w450] -> w32
    tunnel: w31 -> [w449]
    tunnel: [w449] -> w30
    tunnel: [w446] -> w22
    tunnel: w24 -> [w446]
    tunnel: [w445] -> w21
    tunnel: w23 -> [w445]
    tunnel: w11 -> [w444]
    tunnel: w1 -> [w442]
    frame #0 {
      # "Save original data\nto  .csv format"
      n166 = while {
        tunnel: w444 -> [w453]
        tunnel: w442 -> [w451]
        stop <- w452 stop-if-true
        n167 = event shown="[0] \"Save Button\": Value Change" {
          selector: _ -> [_ _]
          dyn-events: _ -> [_ _]
          timeout: _ -> [_ _]
          tunnel: w453 -> [w456 _]
          tunnel: [TRUE TRUE] -> w452
          tunnel: w451 -> [w455 _]
          event "Save Button": Value Change {
            w458 = "%.8f" ("format (%.3f)")
            # "Save original data\nto  .csv format"
            n168 = event-data() -> ()  [unwired: 1 in, 1 out]
            n169 = call "File Dialog"("start path"="Save/Open Link", "pattern (all files)"="*.csv") -> ("selected path"=w454:path)  [unwired: 10 in, 3 out]
            n170 = local write "Save/Open Link"(w454) -> ()
            n171 = Path To String(path=w454) -> (string=w467:string)
            n172 = Match Pattern(string=w467, regular expression=".csv") -> (before substring=w461:string)  [unwired: 1 in, 3 out]
            n173 = Concatenate Strings(w461, "_Hall.csv" ("format (%.3f)")) -> (w464:string)
            n174 = String To Path(string=w464) -> (path=w463:path)
            n175 = call-poly <vilib>:"Write To Spreadsheet File.vi"("delimiter (\\t)"="," ("delimiter (\\t)"), "format (%.3f)"=w458, "2D data"=w456, "file path (dialog if empty)"=w463) -> ()  [unwired: 4 in, 1 out]
            n176 = Concatenate Strings(w461, "_GMR.csv" ("format (%.3f)")) -> (w460:string)
            n177 = String To Path(string=w460) -> (path=w459:path)
            n178 = call-poly <vilib>:"Write To Spreadsheet File.vi"("delimiter (\\t)"="," ("delimiter (\\t)"), "format (%.3f)"=w458, "2D data"=w455, "file path (dialog if empty)"=w459) -> ()  [unwired: 4 in, 1 out]
          }
          event "No Save": Value Change {
            n179 = event-data() -> ()  [unwired: 1 in, 1 out]
          }
        }
      }
      n180 = local write "Back data"(FALSE ("Back data")) -> ()
      n181 = local write "Stop Scan"(FALSE ("Exit")) -> ()
      n182 = local write "Scan"(FALSE ("Scan")) -> ()
    }
  }
  n183 = call <vilib>:"DAQmx Clear Task.vi"("task in"=w22, "error in"=w21) -> ("error out"=w25:errorcluster)  [unwired: 13 in]
  n184 = call <vilib>:"DAQmx Clear Task.vi"("task in"=w32, "error in"=w30) -> ("error out"=w35:errorcluster)  [unwired: 13 in]
  n185 = call <vilib>:"Simple Error Handler.vi"("error in (no error)"=w25) -> ()  [unwired: 4 in, 5 out]
  n186 = call <vilib>:"Simple Error Handler.vi"("error in (no error)"=w35) -> ()  [unwired: 4 in, 5 out]
